vi "Get Time.vi"(8 "error in":errorcluster, 10 "Show Date?":bool) -> (0 "error out":errorcluster, 2 "Time string":string)   [LabVIEW 2021]
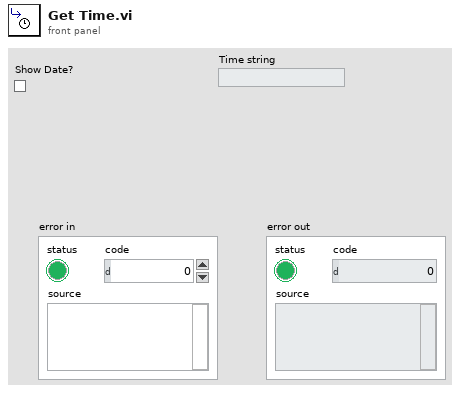
[diagram p1: front panel]
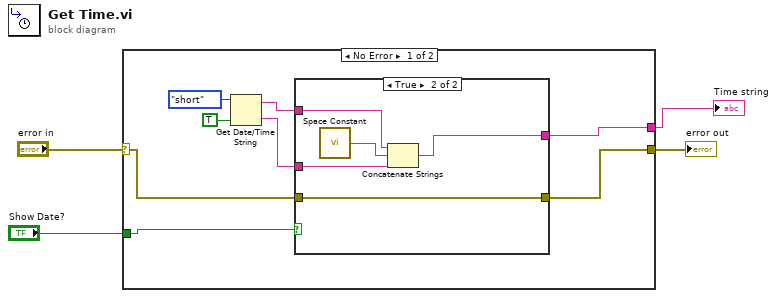
[diagram p0: block diagram]
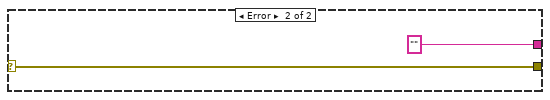
[diagram p3: hidden frame]
diagram:
  n1 = case shown="No Error" "error in" {
    selector: "error in" -> [w7 w21]
    tunnel: [w6 w21] -> w3
    tunnel: [w9 ""] -> w2
    tunnel: "Show Date?" -> [w5 _]
    frame No Error {
      n2 = Get Date/Time String(date format (0)=enum16{"short", "long", "abbreviated"}."short", want seconds? (F)=TRUE) -> (date string=w11:string, time string=w10:string)  [unwired: 1 in]
      n3 = case shown="True" w5 {
        tunnel: w11 -> [_ w19]
        tunnel: w10 -> [w14 w16]
        tunnel: [w14 w17] -> w9
        tunnel: w7 -> [w13 w15]
        tunnel: [w13 w15] -> w6
        frame False {
        }
        frame True {
          n4 = call <vilib>:"Space Constant.vi"() -> ("String"=w18:string)
          n5 = Concatenate Strings(w19, w18, w16) -> (w17:string)
        }
      }
    }
    frame Error {
    }
  }
  "error out" <- w3
  "Time string" <- w2
